vi "4145_Data_Util.vi"() -> ()   [LabVIEW 2014]
uses:
  typedef/4145_GPIB_Com.ctl
  typedef/4145_que_msg.ctl
  typedef/4145 command enum.ctl
  typedef/4145 Spreadsheet data.ctl
  <vilib>/Utility/miscctls.llb/LVRangeTypeDef.ctl
  typedef/4145_X_Axis.ctl
  typedef/4145_Y2_Axis.ctl
  typedef/4145_Y_Axis.ctl
  <vilib>/Utility/file.llb/Write To Spreadsheet File (string).vi
  <vilib>/Utility/file.llb/Write To Spreadsheet File (DBL).vi
panel:
  out "status_op":string
  in  "AdvancedConfig":T1={"X Axis Name"="", "X axis"=TRUE, "X scale"=TRUE, "Is X axis VAR 1?"=FALSE, "X Axis min"=0.0, "X Axis max"=1.0, "Y1 Axis Name"="", "Y1 scale"=TRUE, "Is VAR 2 used?"=FALSE, "# of steps for VAR 2"=0, "Y1 Axis min"=0.0, "Y1 Axis max"=0.01, "Y2 Axis Name"="", "Y2 axis"=FALSE, "Y2 scale"=TRUE, "Y2 Axis min"=0.0, "Y2 Axis max"=0.01} caption="Simple" {"Y2 Axis max" format="%^.3e"; "Y2 Axis min" format="%^.3e"; "Y1 Axis max" format="%^.3e"; "Y1 Axis min" format="%^.3e"; "X Axis max" format="%^.3e"; "X Axis min" format="%^.3e"}
  out "Connected":bool
  out "Accessing?":bool
  out "Status":string
  out "wait":u32
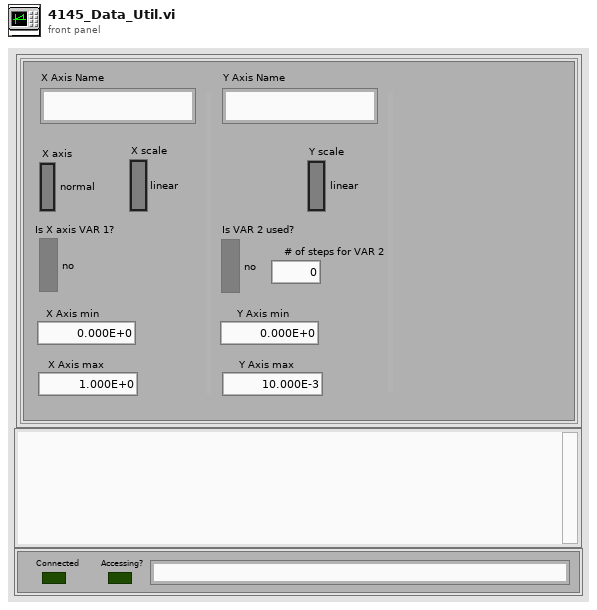
[diagram p1: front panel]
types:
  T1 = cluster{"X Axis Name":string, "X axis":bool, "X scale":bool, "Is X axis VAR 1?":bool, "X Axis min":dbl, "X Axis max":dbl, "Y1 Axis Name":string, "Y1 scale":bool, "Is VAR 2 used?":bool, "# of steps for VAR 2":u16, "Y1 Axis min":dbl, "Y1 Axis max":dbl, "Y2 Axis Name":string, "Y2 axis":bool, "Y2 scale":bool, "Y2 Axis min":dbl, "Y2 Axis max":dbl}
  T2 = typedef "4145 Spreadsheet data.ctl" = cluster{"Spreadsheet formatted":dbl[][], "Spreadsheet header":string[], "graphics plot":cluster{"read data array OUT":dbl[], dbl[]}[], "X Scale.Range":T3, "Y1 Scale.Range ":T3, "Y2 Scale.Range":T3}
  T3 = typedef "LVRangeTypeDef.ctl" = cluster{"Minimum":dbl, "Maximum":dbl, "Increment":dbl, "Minor Increment":dbl, "Start":dbl}
  T4 = typedef "4145_GPIB_Com.ctl" = cluster{"Address_string":string, "timeout ms":u32, "Terminator":string, "LoggerQueue":refnum<queue>}
  T5 = typedef "4145_que_msg.ctl" = cluster{"msg":string, "msg_type":T6}
  T6 = typedef "4145 command enum.ctl" = enum16{"DEFAULT", "INFORMATION", "ERROR", "STATUS", "CAUTION", "WARNING", "OFFLINE", "STOP"}
  T7 = typedef "4145_Y_Axis.ctl" = cluster{"Y1 channel name":string, "Y1 scale":bool, "Y1 min":dbl, "Y1 max":dbl}
  T8 = typedef "4145_Y2_Axis.ctl" = cluster{"Y2 axis":bool, "Y2 channel name":string, "Y2 scale":bool, "Y2 min":dbl, "Y2 max":dbl, "# of steps for VAR 2":u16}
  T9 = typedef "4145_X_Axis.ctl" = cluster{"X axis":bool, "X channel name":string, "X scale":bool, "X min":dbl, "X max":dbl, "Is X axis VAR 1?":bool}
  T10 = enum16{"open", "replace", "create", "open or create", "replace or create", "replace or create with confirmation"}
  T11 = cluster{"error":bool, "code":i32, "source":string}
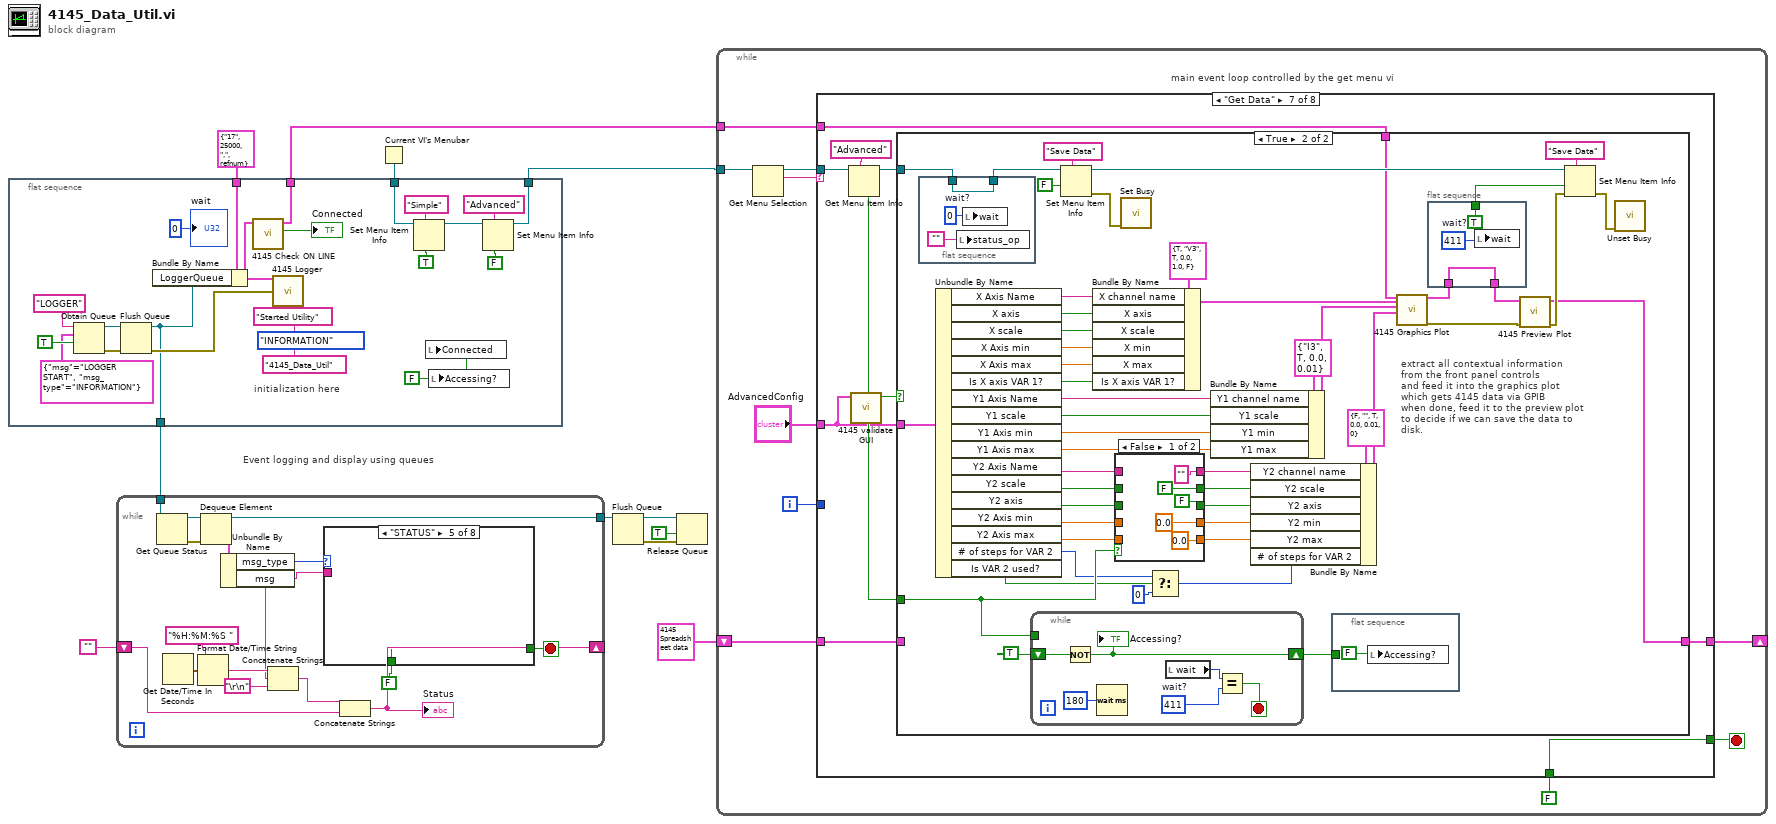
[diagram p0: block diagram]
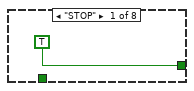
[diagram p2: hidden frame]
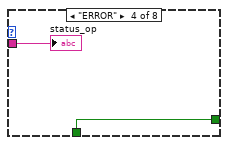
[diagram p5: hidden frame]
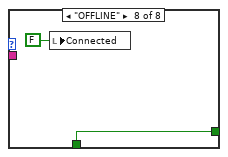
[diagram p8: hidden frame]
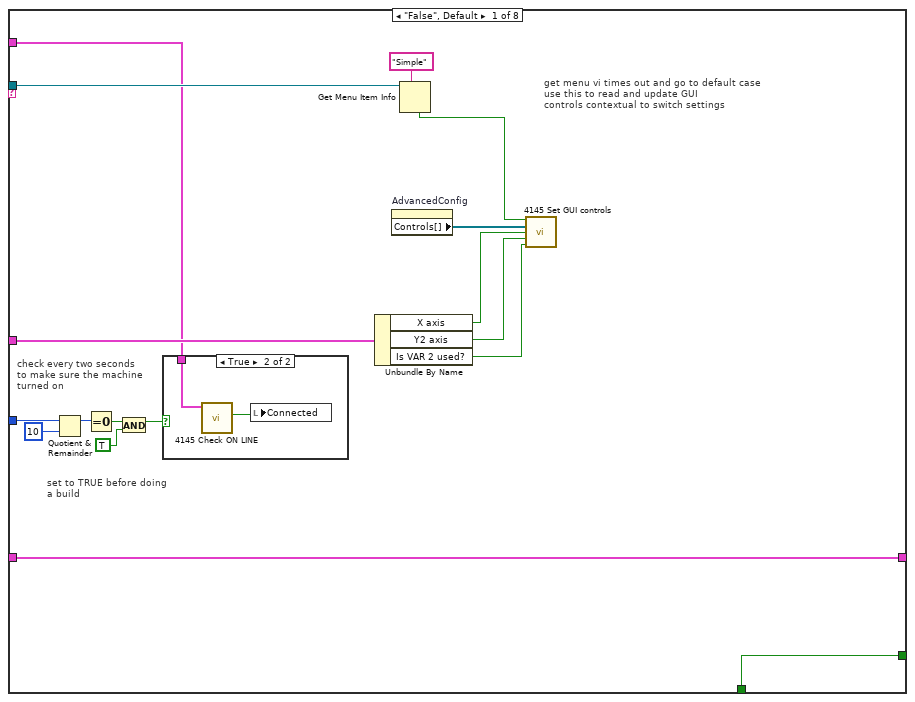
[diagram p9: hidden frame]
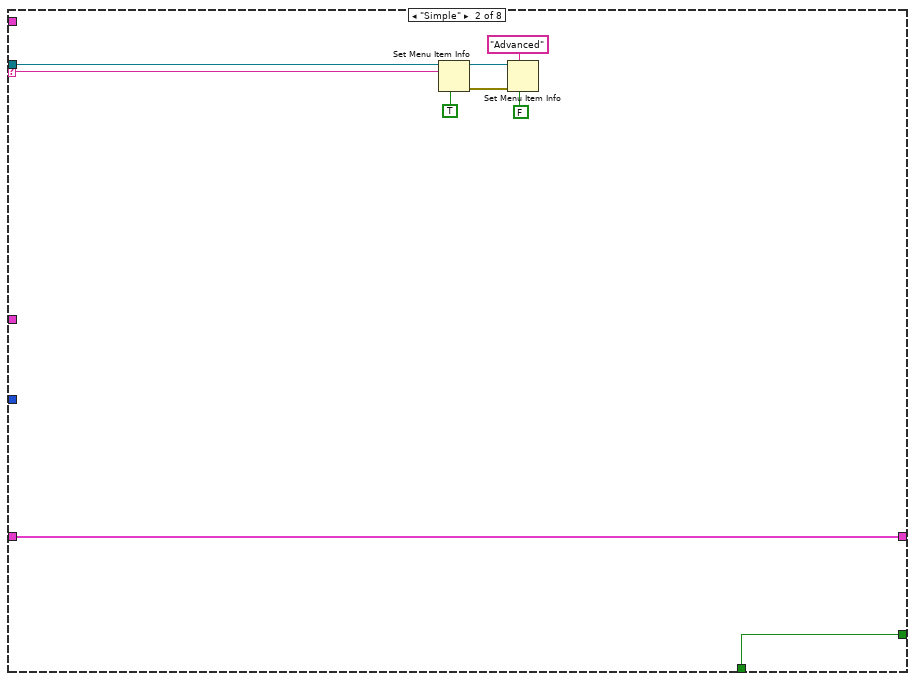
[diagram p11: hidden frame]
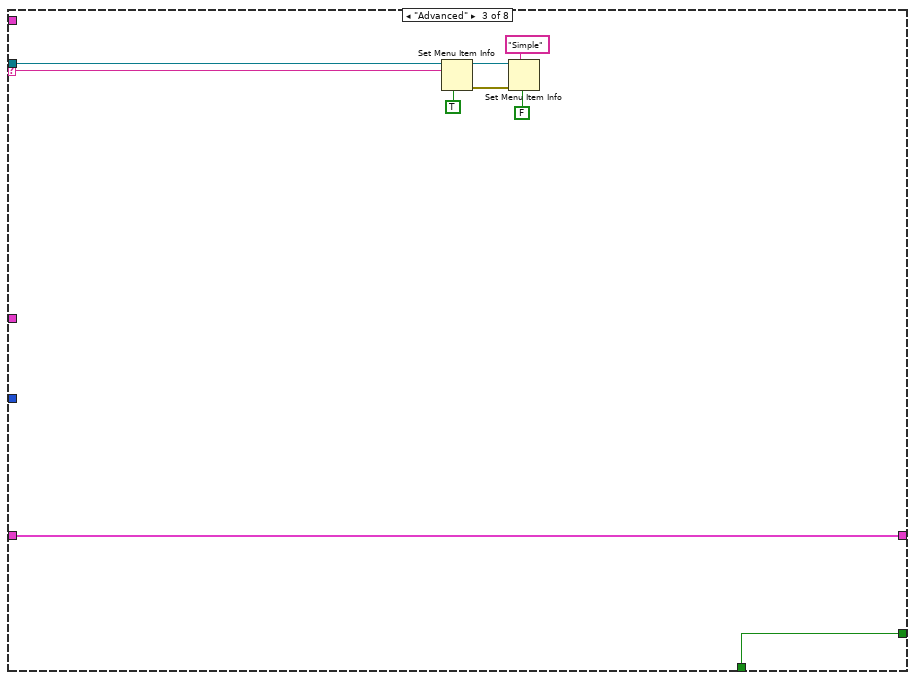
[diagram p12: hidden frame]
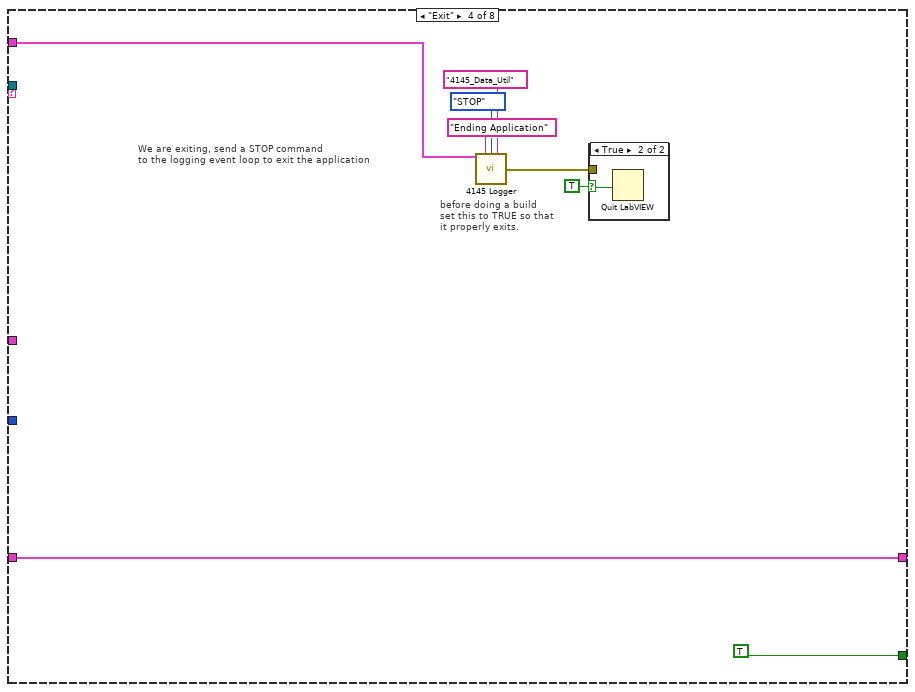
[diagram p13: hidden frame]
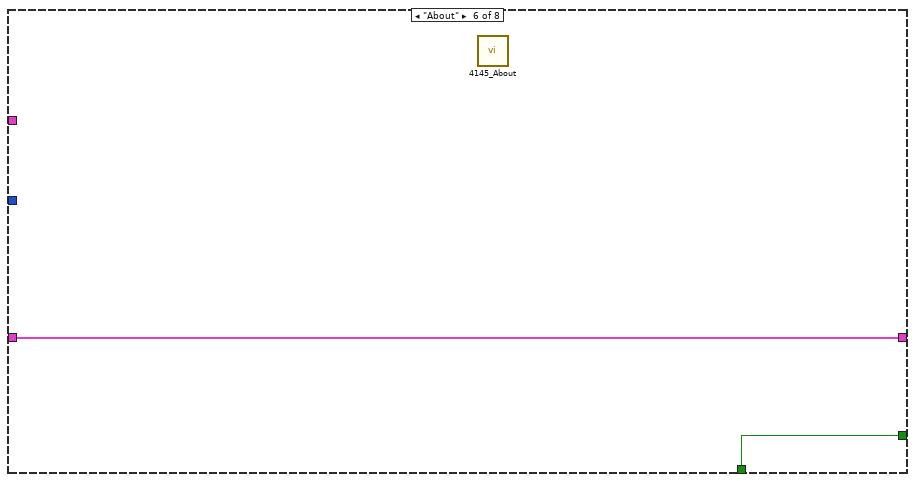
[diagram p16: hidden frame]
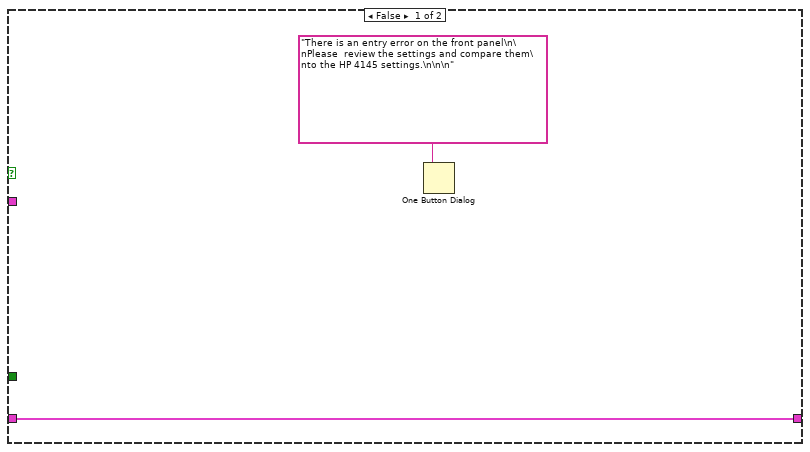
[diagram p17: hidden frame]
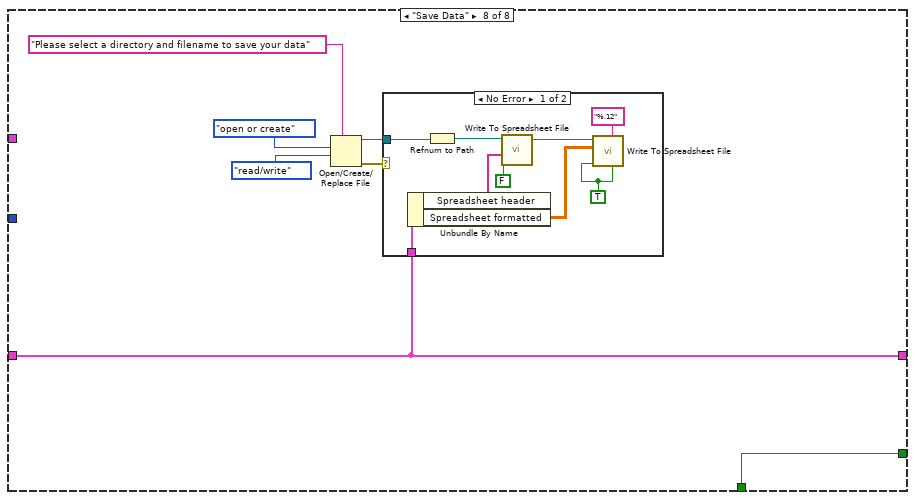
[diagram p19: hidden frame]
diagram:
  # "Event logging and display using queues"
  n1 = flat-sequence {
    tunnel: w11 -> [w12]
    tunnel: [w19] -> w6
    tunnel: T4 {"Address_string"="17", "timeout ms"=25000, "Terminator"=",", "LoggerQueue"=refnum} ("4145_GPIB_COM_IN") -> [w24]
    tunnel: [w29] -> w9
    tunnel: [w13] -> w2
    frame #0 {
      (unwired) 4145_command_enum."INFORMATION" ("msg_type")
      w27 = FALSE ("Accessing?")
      # "initialization here"
      n2 = Obtain Queue(name (unnamed)="LOGGER", element data type=T5 {"msg"="LOGGER START", "msg_type"=enum."INFORMATION"} ("4145_que_msg"), create if not found? (T)=TRUE) -> (queue out=w25:refnum<queue>, error out=w21:errorcluster)  [unwired: 2 in, 1 out]
      n3 = Flush Queue(queue=w25) -> (queue out=w19:refnum<queue>)  [unwired: 1 in, 2 out]
      n4 = Bundle By Name(cluster=w24, "LoggerQueue"=w19) -> (w20:T4)
      n5 = call "4145 Check ON LINE.vi"("4145_GPIB_COM_IN"=w20) -> ("on line?"=→"Connected":bool, "4145_GPIB_COM_OUT"=w29:T4)  [unwired: 7 in, 2 out]
      n6 = call "4145 Logger.vi"("4145_GPIB_COM_ctrl"=w20, "msg"="Started Utility", "origin vi"="4145_Data_Util" ("msg"), "error in (no error)"=w21) -> ()  [unwired: 11 in, 1 out]
      n7 = Set Menu Item Info(6:TRUE ("Visible"), 7:"Simple" ("item tag"), 11:w12) -> (3:w14:refnum<k9>)  [unwired: 4 in, 1 out]
      n8 = local write "Connected"(w27) -> ()
      n9 = local write "Accessing?"(w27) -> ()
      n10 = Set Menu Item Info(6:FALSE ("checked"), 7:"Advanced" ("item tag"), 11:w14) -> (3:w13:refnum<k9>)  [unwired: 4 in, 1 out]
      "wait" <- u32 0 ("wait")
    }
  }
  n11 = while {
    tunnel: w6 -> [w48]
    shift-right: [w34] -> _
    shift-left: "" -> [w35]
    tunnel: [w47] -> w8
    stop <- w44 stop-if-true
    n12 = Get Queue Status(queue=w48) -> (queue out=w42:refnum<queue>, error out=w41:errorcluster)  [unwired: 2 in, 6 out]
    n13 = Get Date/Time In Seconds() -> (seconds since 1Jan1904=w38:timestamp)
    n14 = Format Date/Time String(time format string (%c)="%H:%M:%S ", seconds (now)=w38) -> (date/time string=w39:string)  [unwired: 1 in]
    n15 = Dequeue Element(queue=w42, error in (no error)=w41) -> (queue out=w47:refnum<queue>, element=w46:T5)  [unwired: 1 in, 2 out]
    n16 = Unbundle By Name(w46) -> ("msg_type"=w45:T6, "msg"=w33:string)
    n17 = Concatenate Strings(w39, w33, "\r\n") -> (w36:string)
    n18 = case shown="\"STATUS\"" w45 {
      tunnel: [TRUE w50 w51 w53 w54 w55 w56 w58] -> w44
      tunnel: FALSE -> [_ w50 w51 w53 w54 w55 w56 w58]
      tunnel: w33 -> [_ _ _ w52 _ _ _ _]
      frame "STOP" {
      }
      frame Default {
      }
      frame "INFORMATION" {
      }
      frame "ERROR" {
        "status_op" <- w52
      }
      frame "STATUS" {
      }
      frame "CAUTION" {
      }
      frame "WARNING" {
      }
      frame "OFFLINE" {
        n19 = local write "Connected"(FALSE ("Connected")) -> ()
      }
    }
    n20 = Concatenate Strings(w36, w35) -> (w34:string)
    "Status" <- w34
  }
  n21 = Current VI's Menubar() -> (w11:refnum<k9>)
  n22 = Flush Queue(queue=w8) -> (queue out=w5:refnum<queue>, error out=w4:errorcluster)  [unwired: 1 in, 1 out]
  n23 = Release Queue(queue=w5, force destroy? (F)=TRUE, error in (no error)=w4) -> ()  [unwired: 3 out]
  n24 = while {
    tunnel: w2 -> [w68]
    shift-right: [w61] -> _
    shift-left: T2 {"Spreadsheet formatted"=[], "Spreadsheet header"=[], "graphics plot"=[], "X Scale.Range"={"Minimum"=0.0, "Maximum"=0.0, "Increment"=0.0, "Minor Increment"=0.0, "Start"=0.0}, "Y1 Scale.Range "={"Minimum"=0.0, "Maximum"=0.0, "Increment"=0.0, "Minor Increment"=0.0, "Start"=0.0}, "Y2 Scale.Range"={"Minimum"=0.0, "Maximum"=0.0, "Increment"=0.0, "Minor Increment"=0.0, "Start"=0.0}} ("Spreadsheet data") -> [w62]
    tunnel: w9 -> [w60]
    i -> [w59]
    stop <- w66 stop-if-true
    # "main event loop controlled by the get menu vi"
    n25 = Get Menu Selection(0:w68) -> (5:w64:refnum<k9>, 6:w67:string)  [unwired: 3 in, 3 out]
    n26 = case shown="\"Get Data\"" w67 {
      selector: w67 -> [_ w88 w97 _ _ _ _ _]
      tunnel: [w85 w96 w105 TRUE w116 w118 w128 w209] -> w66
      tunnel: FALSE -> [w85 w96 w105 _ w116 w118 w128 w209]
      tunnel: w64 -> [w84 w95 w102 _ _ _ w122 _]
      tunnel: "AdvancedConfig" -> [w82 _ _ _ _ _ w119 _]
      tunnel: w62 -> [w81 w90 w99 w113 w115 w117 w124 w208]
      tunnel: [w81 w90 w99 w113 w115 w117 w127 w208] -> w61
      tunnel: w60 -> [w73 _ _ w111 _ _ w126 _]
      tunnel: w59 -> [w76 _ _ _ _ _ _ _]
      frame "False", Default {
        # "check every two seconds\nto make sure the machine \nturned on"
        # "set to TRUE before doing \na build"
        # "get menu vi times out and go to default case \nuse this to read and update GUI \ncontrols contextual to switch settings"
        n27 = Quotient & Remainder(x=w76, y=10) -> (x-y*floor(x/y)=w74:i32)  [unwired: 1 out]
        n28 = Equal To 0?(x=w74) -> (x = 0?=w72:bool)
        n29 = And(x=w72, y=TRUE) -> (x .and. y?=w71:bool)
        n30 = case shown="True" w71 {
          tunnel: w73 -> [_ w87]
          frame False {
          }
          frame True {
            n31 = call "4145 Check ON LINE.vi"("4145_GPIB_COM_IN"=w87) -> ("on line?"=w86:bool)  [unwired: 7 in, 3 out]
            n32 = local write "Connected"(w86) -> ()
          }
        }
        n33 = Unbundle By Name(w82) -> ("X axis"=w78:bool, "Y2 axis"=w77:bool, "Is VAR 2 used?"=w69:bool)
        n34 = property on="AdvancedConfig" class="Clust (strict)"() -> ("Controls[]"=w79:refnum<vi>[])  [unwired: 2 in, 2 out]
        n35 = Get Menu Item Info(7:"Simple" ("item tag"), 11:w84) -> (4:w80:bool)  [unwired: 1 in, 6 out]
        n36 = call "4145 Set GUI controls.vi"("Simple/Advanced Checked?"=w80, "Panel Controls[]"=w79, "X axis"=w78, "Y2 axis"=w77, "Is VAR 2 used?"=w69) -> ()  [unwired: 11 in]
      }
      frame "Simple" {
        n37 = Set Menu Item Info(6:TRUE ("Visible"), 7:w88, 11:w95) -> (0:w89:errorcluster, 3:w94:refnum<k9>)  [unwired: 4 in]
        n38 = Set Menu Item Info(6:FALSE ("checked"), 7:"Advanced" ("item tag"), 8:w89, 11:w94) -> ()  [unwired: 3 in, 2 out]
      }
      frame "Advanced" {
        n39 = Set Menu Item Info(6:TRUE ("checked"), 7:w97, 11:w102) -> (0:w98:errorcluster, 3:w104:refnum<k9>)  [unwired: 4 in]
        n40 = Set Menu Item Info(6:FALSE ("checked"), 7:"Simple" ("item tag"), 8:w98, 11:w104) -> ()  [unwired: 3 in, 2 out]
      }
      frame "Exit" {
        # "before doing a build\nset this to TRUE so that\nit properly exits."
        # "We are exiting, send a STOP command\nto the logging event loop to exit the application"
        n41 = call "4145 Logger.vi"("4145_GPIB_COM_ctrl"=w111, "msg"="Ending Application", "msg_type"=4145_command_enum."STOP", "origin vi"="4145_Data_Util" ("msg")) -> ("error out"=w106:errorcluster)  [unwired: 11 in]
        n42 = case shown="True" TRUE {
          selector: TRUE -> [_ w114]
          tunnel: w106 -> [_ _]
          frame False {
          }
          frame True {
            n43 = Quit LabVIEW(quit? (T)=w114) -> ()
          }
        }
      }
      frame "Options" {
      }
      frame "About" {
        n44 = call "4145_About.vi"() -> ()  [unwired: 12 in]
      }
      frame "Get Data" {
        n45 = Get Menu Item Info(7:"Advanced" ("item tag"), 11:w122) -> (3:w121:refnum<k9>, 4:w120:bool)  [unwired: 1 in, 5 out]
        n46 = call "4145 validate GUI.vi"("advanced?"=w120, "AdvancedConfig"=w119) -> ("valid"=w125:bool)  [unwired: 8 in, 1 out]
        n47 = case shown="True" w125 {
          tunnel: [w130 w135] -> w127
          tunnel: w126 -> [_ w142]
          tunnel: w119 -> [_ w141]
          tunnel: w124 -> [w130 _]
          tunnel: w121 -> [_ w139]
          tunnel: w120 -> [_ w140]
          frame False {
            n48 = One Button Dialog(message="There is an entry error on the front panel\n\nPlease  review the settings and compare them\nto the HP 4145 settings.\n\n\n") -> ()  [unwired: 1 in, 1 out]
          }
          frame True {
            # "extract all contextual information \nfrom the front panel controls\nand feed it into the graphics plot\nwhich gets 4145 data via GPIB\nwhen done, feed it to the preview plot\nto decide if we can save the data to\ndisk."
            n49 = flat-sequence {
              tunnel: w139 -> [w185]
              tunnel: [w185] -> w138
              frame #0 {
                w186 = u32 0  # wait?
                n50 = local write "status_op"("") -> ()
                n51 = local write "wait"(w186) -> ()
              }
            }
            n52 = Unbundle By Name(w141) -> ("X Axis Name"=w152:string, "X axis"=w151:bool, "X scale"=w150:bool, "X Axis min"=w149:dbl, "X Axis max"=w148:dbl, "Is X axis VAR 1?"=w147:bool, "Y1 Axis Name"=w146:string, "Y1 scale"=w145:bool, "Y1 Axis min"=w144:dbl, "Y1 Axis max"=w143:dbl, "Y2 Axis Name"=w153:string, "Y2 scale"=w154:bool, "Y2 axis"=w155:bool, "Y2 Axis min"=w156:dbl, "Y2 Axis max"=w157:dbl, "# of steps for VAR 2"=w134:u16, "Is VAR 2 used?"=w132:bool)
            n53 = while {
              tunnel: w140 -> [_]
              shift-right: [w187] -> w158
              shift-left: TRUE -> [w188]
              stop <- w189 stop-if-true
              w190 = u32 411  # wait?
              n54 = Not(x=w188) -> (.not. x?=w187:bool)
              "Accessing?" <- w187
              n55 = Wait (ms)(milliseconds to wait=u32 180) -> ()  [unwired: 1 out]
              n56 = local read "wait"() -> (w191:u32)
              n57 = Equal?(x=w191, y=w190) -> (x = y?=w189:bool)
            }
            n58 = Set Menu Item Info(7:"Save Data", 9:FALSE ("enabled"), 11:w138) -> (0:w163:errorcluster, 3:w165:refnum<k9>)  [unwired: 4 in]
            n59 = Bundle By Name(cluster=T9 {"X axis"=TRUE, "X channel name"="V3", "X scale"=TRUE, "X min"=0.0, "X max"=1.0, "Is X axis VAR 1?"=FALSE} ("4145_X_Axis_IN"), "X channel name"=w152, "X axis"=w151, "X scale"=w150, "X min"=w149, "X max"=w148, "Is X axis VAR 1?"=w147) -> (w176:T9)
            n60 = case shown="False" w140 {
              tunnel: ["" ("Y2 Axis Name") w198] -> w173
              tunnel: [0.0 ("Y2 Axis min") w201] -> w172
              tunnel: [0.0 ("Y2 Axis max") w202] -> w171
              tunnel: [FALSE ("Y2 scale") w199] -> w170
              tunnel: [FALSE ("Y2 axis") w200] -> w169
              tunnel: w157 -> [_ w202]
              tunnel: w156 -> [_ w201]
              tunnel: w155 -> [_ w200]
              tunnel: w154 -> [_ w199]
              tunnel: w153 -> [_ w198]
              frame False {
              }
              frame True {
              }
            }
            n61 = call <vilib>:"Set Busy.vi"("error in (no error)"=w163) -> ()  [unwired: 9 in, 2 out]
            n62 = Select(t=w134, s=w132, f=u16 0) -> (s? t:f=w133:u16)
            n63 = Bundle By Name(cluster=T7 {"Y1 channel name"="I3", "Y1 scale"=TRUE, "Y1 min"=0.0, "Y1 max"=0.01} ("4145_Y_Axis_IN"), "Y1 channel name"=w146, "Y1 scale"=w145, "Y1 min"=w144, "Y1 max"=w143) -> (w174:T7)
            n64 = Bundle By Name(cluster=T8 {"Y2 axis"=FALSE, "Y2 channel name"="", "Y2 scale"=TRUE, "Y2 min"=0.0, "Y2 max"=0.01, "# of steps for VAR 2"=0} ("4145_Y2_Axis_IN"), "Y2 channel name"=w173, "Y2 scale"=w170, "Y2 axis"=w169, "Y2 min"=w172, "Y2 max"=w171, "# of steps for VAR 2"=w133) -> (w175:T8)
            n65 = flat-sequence {
              tunnel: w158 -> [_]
              frame #0 {
                n66 = local write "Accessing?"(FALSE ("Accessing?")) -> ()
              }
            }
            n67 = call "4145 Graphics Plot.vi"("4145_GPIB_COM_IN"=w142, "4145_X_Axis_IN"=w176, "4145_Y_Axis_IN"=w174, "4145_Y2_Axis_IN"=w175) -> ("Spreadsheet data"=w137:T2, "error out"=w161:T11)  [unwired: 13 in, 1 out]
            n68 = flat-sequence {
              tunnel: [TRUE] -> w160
              tunnel: w137 -> [w181]
              tunnel: [w181] -> w136
              frame #0 {
                w183 = u32 411  # wait?
                n69 = local write "wait"(w183) -> ()
              }
            }
            n70 = call "4145 Preview Plot.vi"("error in (no error)"=w161, "Spreadsheet data IN"=w136) -> ("error out"=w164:errorcluster, "Spreadsheet data OUT"=w135:T2)  [unwired: 8 in]
            n71 = Set Menu Item Info(7:"Save Data", 8:w164, 9:w160, 11:w165) -> (0:w162:errorcluster)  [unwired: 3 in, 1 out]
            n72 = call <vilib>:"Unset Busy.vi"("error in (no error)"=w162) -> ()  [unwired: 10 in, 1 out]
          }
        }
      }
      frame "Save Data" {
        n73 = Open/Create/Replace File(prompt="Please select a directory and filename to save your data", operation (0:open)=T10."open or create", access (0:read/write)=enum16{"read/write", "read-only", "write-only"}."read/write") -> (refnum out=w206:refnum<file>, error out=w207:errorcluster)  [unwired: 3 in, 1 out]
        n74 = case shown="No Error" w207 {
          tunnel: w208 -> [w216 _]
          tunnel: w206 -> [w211 _]
          frame No Error {
            w212 = TRUE
            n75 = Unbundle By Name(w216) -> ("Spreadsheet header"=w214:string[], "Spreadsheet formatted"=w215:dbl[][])
            n76 = Refnum to Path(1:w211) -> (0:w210:path)
            n77 = call-poly <vilib>:"Write To Spreadsheet File.vi"("append to file? (new file:F)"=FALSE, "1D data"=w214, "file path (dialog if empty)"=w210) -> ("new file path (Not A Path if cancelled)"=w217:path)  [unwired: 5 in]
            n78 = call-poly <vilib>:"Write To Spreadsheet File.vi"("transpose? (no:F)"=w212, "format (%.3f)"="%.12", "append to file? (new file:F)"=w212, "2D data"=w215, "file path (dialog if empty)"=w217) -> ()  [unwired: 3 in, 1 out]
          }
          frame Error {
          }
        }
      }
    }
  }
